vi "Populate Connection Destination List.vi"(6 "initial Destination":string, 7 "Source":string, 8 "Alias Mappings by Module":T1[](array[typedef]), 9 "Possible Connections":T3(array[cluster]), 10 "Module Index":i32, 11 "Destination Reference":refnum<vi>) -> (2 "Endpoint List":string[](array[string]), 3 "Alias List":string[](array[string]))   [LabVIEW 2017, in "Routing and Faulting System Explorer.lvlib"]
uses:
  Routing and Faulting System Explorer.lvlib
  Shared/Routing and Faulting Hardware API/Types/Possible Connections for Endpoint.ctl
  Alias Map by Module.ctl
  Shared/Routing and Faulting Hardware API/Routing and Faulting Hardware API.lvlib
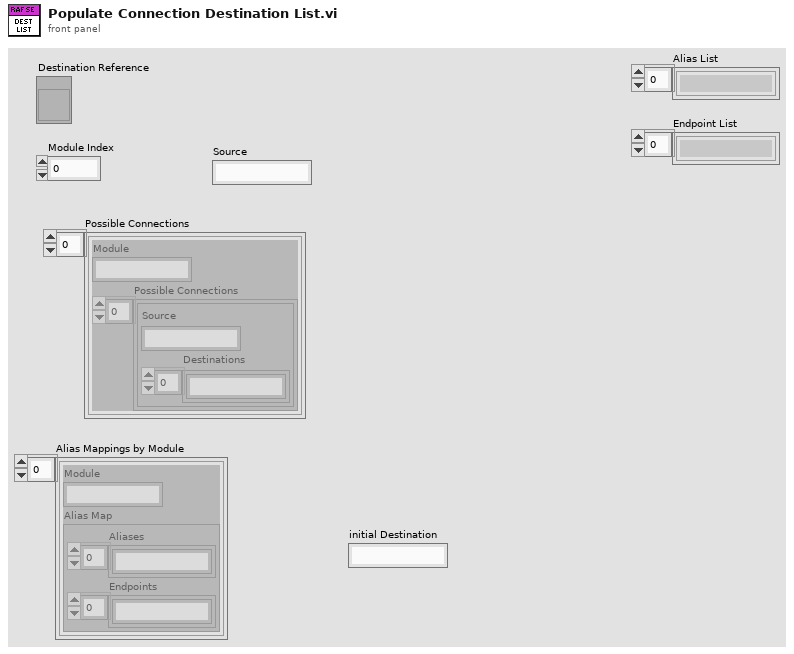
[diagram p1: front panel]
types:
  T1 = typedef "Routing and Faulting System Explorer.lvlib/Alias Map by Module.ctl" = cluster{"Module":string, "Alias Map":cluster{"Aliases":string[], "Endpoints":string[]}}
  T2 = typedef "Routing and Faulting Hardware API.lvlib/Possible Connections for Endpoint.ctl" = cluster{"Source":string, "Destinations":string[]}
  T3 = cluster{"Module":string, "Possible Connections":T2[]}[]
  T4 = cluster{"Module":string, "Possible Connections":T2[]}
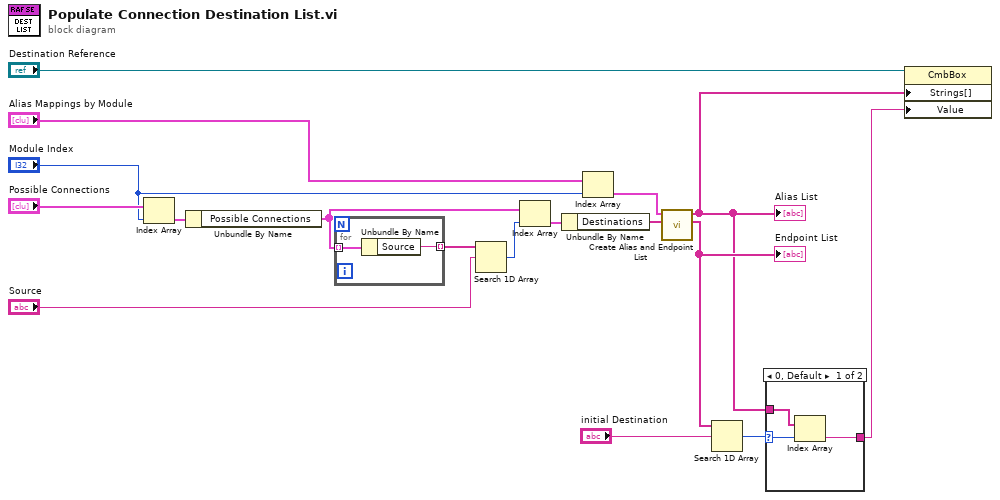
[diagram p0: block diagram]
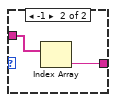
[diagram p2: hidden frame]
diagram:
  n1 = Index Array(array="Possible Connections", index="Module Index") -> (element=w16:T4)
  n2 = Unbundle By Name(w16) -> ("Possible Connections"=w17:T2[])
  n3 = for {
    tunnel: [w19] -> w15 mode=indexing
    tunnel: w17 -> [w18] mode=indexing
    n4 = Unbundle By Name(w18) -> ("Source"=w19:string)
  }
  n5 = Search 1D Array(1D array=w15, element="Source") -> (index of element=w7:i32)  [unwired: 1 in]
  n6 = Index Array(array=w17, index=w7) -> (element=w8:T2)
  n7 = Unbundle By Name(w8) -> ("Destinations"=w12:string[])
  n8 = Index Array(array="Alias Mappings by Module", index="Module Index") -> (element=w11:T1)
  n9 = call "Create Alias and Endpoint List.vi"("Endpoints"=w12, "Alias Mapping"=w11) -> ("Endpoint List"=w3:string[], "Alias List"=w2:string[])  [unwired: 8 in]
  "Endpoint List" <- w3
  "Alias List" <- w2
  n10 = Search 1D Array(1D array=w3, element="initial Destination") -> (index of element=w4:i32)  [unwired: 1 in]
  n11 = case shown="0, Default" w4 {
    selector: w4 -> [w22 _]
    tunnel: w2 -> [w21 w24]
    tunnel: [w20 w23] -> w1
    frame 0, Default {
      n12 = Index Array(array=w21, index=w22) -> (element=w20:string)
    }
    frame -1 {
      n13 = Index Array(array=w24) -> (element=w23:string)  [unwired: 1 in]
    }
  }
  n14 = property on="Property Node" class="CmbBox"(reference="Destination Reference", "Strings[]"=w2, "Value"=w1) -> ()  [unwired: 1 in, 2 out]
